vi "Simulator Load TestSets in Tree.vi"(8 "error in (no error)":errorcluster, 10 "Simulated Configurations":T1[](array[typedef]) {"Calibration Date" format="%.2f"; "Parameters"."TX2pmax" format="%.1f"; "Parameters"."TX1pmax" format="%.1f"; "Parameters"."RXstop" format="%.1f"; "Parameters"."RXstart" format="%.1f"; "Parameters"."TX2stop" format="%.1f"; "Parameters"."TX2start" format="%.1f"; "Parameters"."TX1stop" format="%.1f"; "Parameters"."TX1start" format="%.1f"}, 11 "Tree Control Reference":refnum<vi>) -> (0 "error out":errorcluster, 2 "Populated Configurations":T1[](array[typedef]) {"Calibration Date" format="%.2f"; "Parameters"."TX2pmax" format="%.1f"; "Parameters"."TX1pmax" format="%.1f"; "Parameters"."RXstop" format="%.1f"; "Parameters"."RXstart" format="%.1f"; "Parameters"."TX2stop" format="%.1f"; "Parameters"."TX2start" format="%.1f"; "Parameters"."TX1stop" format="%.1f"; "Parameters"."TX1start" format="%.1f"})   [LabVIEW 2011]
uses:
  PIM Configuration.ctl
  PIM Interface Language.ctl
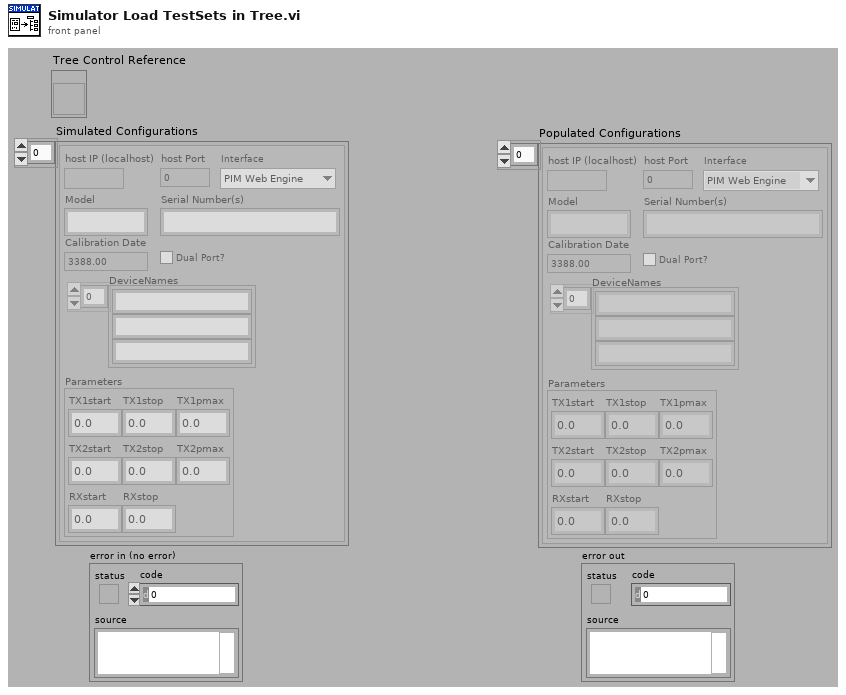
[diagram p1: front panel]
types:
  T1 = typedef "PIM Configuration.ctl" = cluster{"host IP (localhost)":string, "host Port":u16, "Model":string, "Serial Number(s)":string, "Calibration Date":dbl, "Dual Port?":bool, "DeviceNames":string[], "Parameters":cluster{"TX1start":dbl, "TX1stop":dbl, "TX1pmax":dbl, "TX2start":dbl, "TX2stop":dbl, "TX2pmax":dbl, "RXstart":dbl, "RXstop":dbl}, "Interface":T2}
  T2 = typedef "PIM Interface Language.ctl" = enum16{"PIM Web Engine", "PIM HW Engine"}
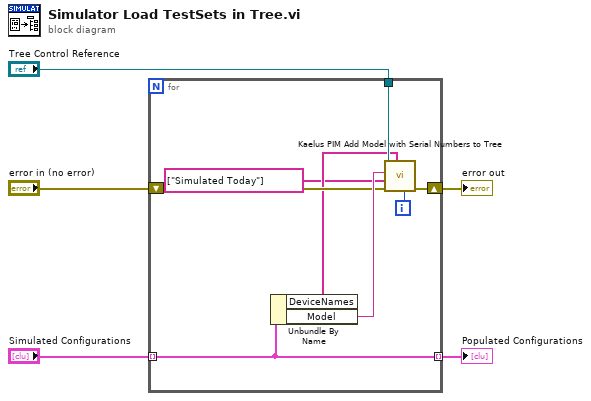
[diagram p0: block diagram]
diagram:
  n1 = for {
    shift-right: [w13] -> w4
    shift-left: "error in (no error)" -> [w9]
    tunnel: "Tree Control Reference" -> [w12]
    tunnel: [w7] -> w2 mode=indexing
    tunnel: "Simulated Configurations" -> [w7] mode=indexing
    i -> [w11]
    n2 = Unbundle By Name(w7) -> ("DeviceNames"=w8:string[], "Model"=w10:string)
    n3 = call "Kaelus PIM Add Model with Serial Numbers to Tree.vi"("Instrument Index"=w11, "Model Serial Numbers"=w8, "error in (no error)"=w9, "Model Descriptive Columns"=string[] ["Simulated Today"], "Model Name"=w10, "Tree Control Reference"=w12) -> ("error out"=w13:errorcluster)  [unwired: 5 in]
  }
  "error out" <- w4
  "Populated Configurations" <- w2
